vi "Material-Line1-TestMain.vi"(8 "error in (no error)":errorcluster, 11 "Material-RunTest in":refnum<class "Material-RunTest.lvclass">) -> (0 "error out":errorcluster, 3 "Material-RunTest out":refnum<class "Material-RunTest.lvclass">)   [LabVIEW 2013, in "Material-RunTest.lvclass"]
uses:
  Material-RunTest.lvclass
  Material-RunTest.lvclass/Material-RunTest.ctl
  Motion Control/Motion-ControlAll.lvclass
  <vilib>/addons/_LabVIEW Style Book/Utilities/Style Book Utilities.lvlib
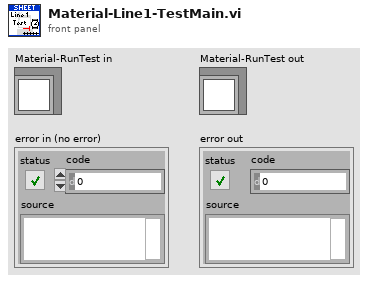
[diagram p1: front panel]
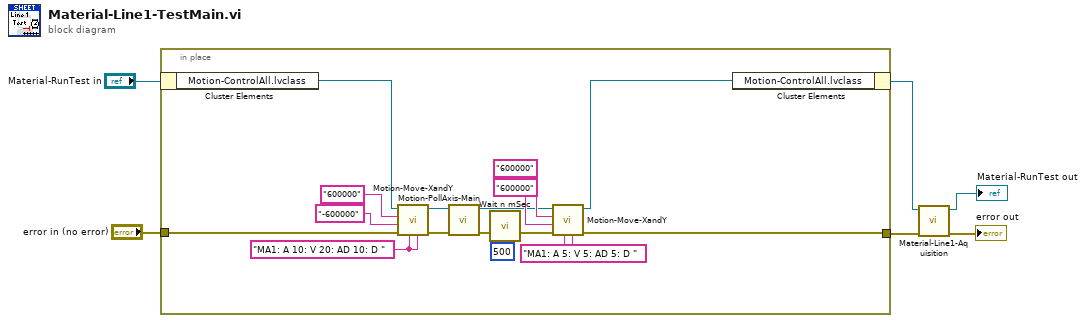
[diagram p0: block diagram]
diagram:
  n1 = in-place {
    in-place-border: "error in (no error)" -> [w22]
    in-place-border: [w7] -> w4
    w11 = "MA1: A 10: V 20: AD 10: D " ("concatenated string")
    w12 = "MA1: A 5: V 5: AD 5: D " ("concatenated string")
    n2 = in-place-cluster #1("Material-RunTest in") -> ("Motion-ControlAll.lvclass"=w21:refnum<class "Motion-ControlAll.lvclass">)
    n3 = call "Motion-Move-XandY.vi"("Y Drive Acc/Speed/Velocity"=w11, "X Drive Acc/Speed/Velocity"=w11, "error in (no error)"=w22, "X Coordinates"="-600000", "Y Coordinates"="600000", "Motion-ControlAll in"=w21) -> ("error out"=w19:errorcluster, "Motion-ControlAll out"=w20:refnum<class "Motion-ControlAll.lvclass">)  [unwired: 4 in]
    n4 = call "Motion-PollAxis-Main.vi"("error in (no error)"=w19, "Motion-ControlAll in"=w20) -> ("error out"=w10:errorcluster, "Motion-ControlAll out"=w14:refnum<class "Motion-ControlAll.lvclass">)  [unwired: 8 in]
    n5 = call <vilib>:"Wait n mSec.vi"("error in (no error)"=w10, "Milliseconds to Wait (500)"=u32 500) -> ("error out"=w9:errorcluster)  [unwired: 13 in]
    n6 = call "Motion-Move-XandY.vi"("Y Drive Acc/Speed/Velocity"=w12, "X Drive Acc/Speed/Velocity"=w12, "error in (no error)"=w9, "X Coordinates"="600000", "Y Coordinates"="600000", "Motion-ControlAll in"=w14) -> ("error out"=w7:errorcluster, "Motion-ControlAll out"=w13:refnum<class "Motion-ControlAll.lvclass">)  [unwired: 4 in]
    n7 = in-place-cluster #1("Motion-ControlAll.lvclass"=w13) -> (w2:refnum<class "Material-RunTest.lvclass">)
  }
  n8 = call "Material-Line1-Aquisition.vi"("error in (no error)"=w4, "Material-RunTest in"=w2) -> ("error out"=→"error out":errorcluster, "Material-RunTest out"=→"Material-RunTest out":refnum<class "Material-RunTest.lvclass">)  [unwired: 8 in]
